vi "GetIntValue.vi"(0 "nInputHandle":u64, 5 "strName":string, 11 "error in (no error)":errorcluster) -> (4 "nOutputHandle":u64, 6 "nCurValue":i32, 8 "pstIntValue":T1, 10 "GX_STATUS":i32, 15 "error out":errorcluster)   [LabVIEW 2016, in "GxLVLib.lvlib"]
uses:
  GxLVLib.lvlib
  GxIAPI.dll
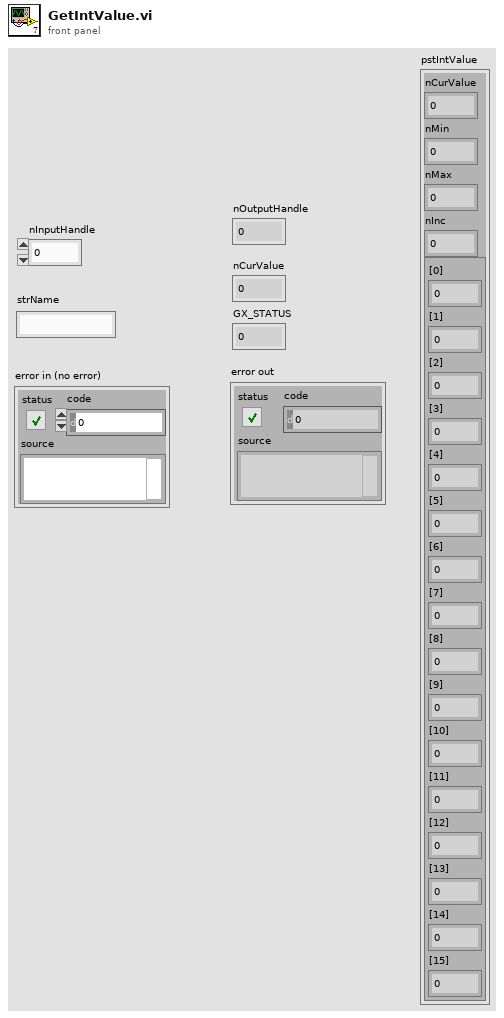
[diagram p1: front panel]
types:
  T1 = cluster{"nCurValue":i64, "nMin":i64, "nMax":i64, "nInc":i64, cluster{"[0]":i32, "[1]":i32, "[2]":i32, "[3]":i32, "[4]":i32, "[5]":i32, "[6]":i32, "[7]":i32, "[8]":i32, "[9]":i32, "[10]":i32, "[11]":i32, "[12]":i32, "[13]":i32, "[14]":i32, "[15]":i32}}
  T2 = cluster{"[0]":i32, "[1]":i32, "[2]":i32, "[3]":i32, "[4]":i32, "[5]":i32, "[6]":i32, "[7]":i32, "[8]":i32, "[9]":i32, "[10]":i32, "[11]":i32, "[12]":i32, "[13]":i32, "[14]":i32, "[15]":i32}
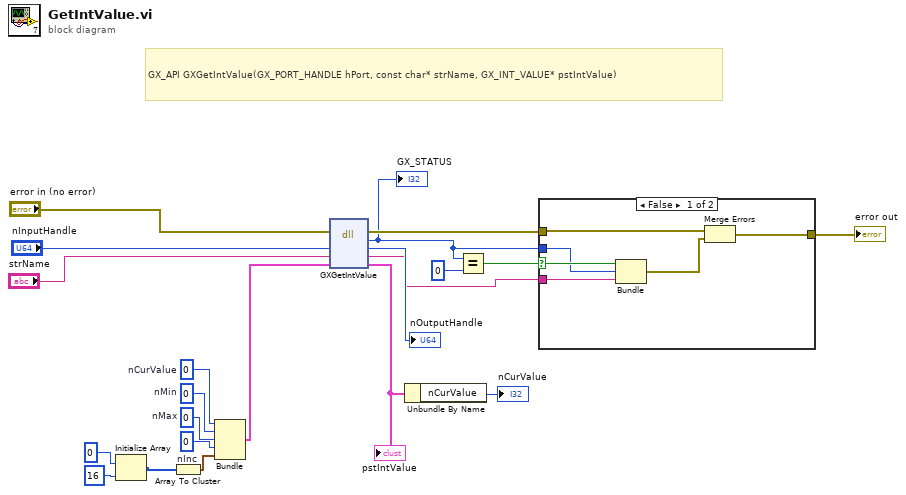
[diagram p0: block diagram]
diagram:
  w18 = i64 0  # nInc
  w19 = i64 0  # nMax
  w20 = i64 0  # nMin
  w21 = i64 0  # nCurValue
  # "GX_API GXGetIntValue(GX_PORT_HANDLE hPort, const char* strName, GX_INT_VALUE* pstIntValue)"
  n1 = Initialize Array(0, 16) -> (w8:i32[])
  n2 = Array To Cluster(array=w8) -> (cluster=w9:T2)
  n3 = Bundle("nCurValue"=w21, "nMin"=w20, "nMax"=w19, "nInc"=w18, w9) -> (w15:T1)  [unwired: 1 in]
  n4 = dll-call lib="GxIAPI.dll" fn="GXGetIntValue"(error in="error in (no error)", "hDevice"="nInputHandle", "strName"="strName", "pstIntValue"=w15) -> (error out=w13:errorcluster, "GX_STATUS"=w4:i32, "hDevice"=→"nOutputHandle":i64, "strName"=w10:string, "pstIntValue"=w7:T1)  [unwired: 2 in, 1 out]
  "GX_STATUS" <- w4
  "pstIntValue" <- w7
  n5 = Unbundle By Name(w7) -> ("nCurValue"=→"nCurValue":i64)
  n6 = Equal?(x=w4, y=0) -> (x = y?=w11:bool)
  n7 = case shown="False" w11 {
    selector: w11 -> [w24 _]
    tunnel: w13 -> [w27 w28]
    tunnel: [w26 w28] -> w5
    tunnel: w4 -> [w23 _]
    tunnel: w10 -> [w22 _]
    frame False {
      n8 = Bundle(w24, "GX_STATUS"=w23, "strName"=w22) -> (w25:cluster{bool, "GX_STATUS":i32, "strName":string})  [unwired: 1 in]
      n9 = Merge Errors(w27, w25) -> (w26:errorcluster)
    }
    frame True {
    }
  }
  "error out" <- w5
